vi "LVClass_ClosedLoopSmoothing_GetData.vi"(0 "ClosedLoopSmoothing in":refnum<class "ClosedLoopSmoothing.lvclass">, 11 "error in (no error)":errorcluster) -> (4 "ClosedLoopSmoothing out":refnum<class "ClosedLoopSmoothing.lvclass">, 6 "CLoopSmoothingParams":T1, 15 "error out":errorcluster)   [LabVIEW 2020, in "ClosedLoopSmoothing.lvclass"]
doc: "Get closed loop smoothing parameters.\n\n<B>smoothing_paramsIn</B> : Closed Loop smoothing params object.\n<B>smoothing_paramsOut</B> : Closed Loop smoothing params object.\n<B>low_gain_factor</B> : lowest value for gain factor\n<B>high_gain_factor</B> : highest value for gain factor\n<B>low_amplitude</B> : lowest amplitude value before switching to linear behavior\n<B>high_amplitude</B> : highest amplitude value where linear behavior stops"
uses:
  ClosedLoopSmoothing.lvclass
  ClosedLoopSmoothingParameters.ctl
  ClosedLoopSmoothing.lvclass/ClosedLoopSmoothing.ctl
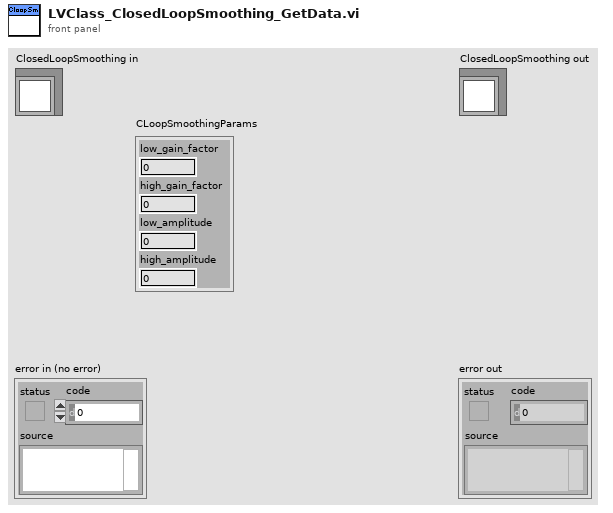
[diagram p1: front panel]
types:
  T1 = typedef "ClosedLoopSmoothingParameters.ctl" = cluster{"low_gain_factor":sgl, "high_gain_factor":sgl, "low_amplitude":i32, "high_amplitude":i32}
  T2 = typedef "ClassID.ctl" = i64
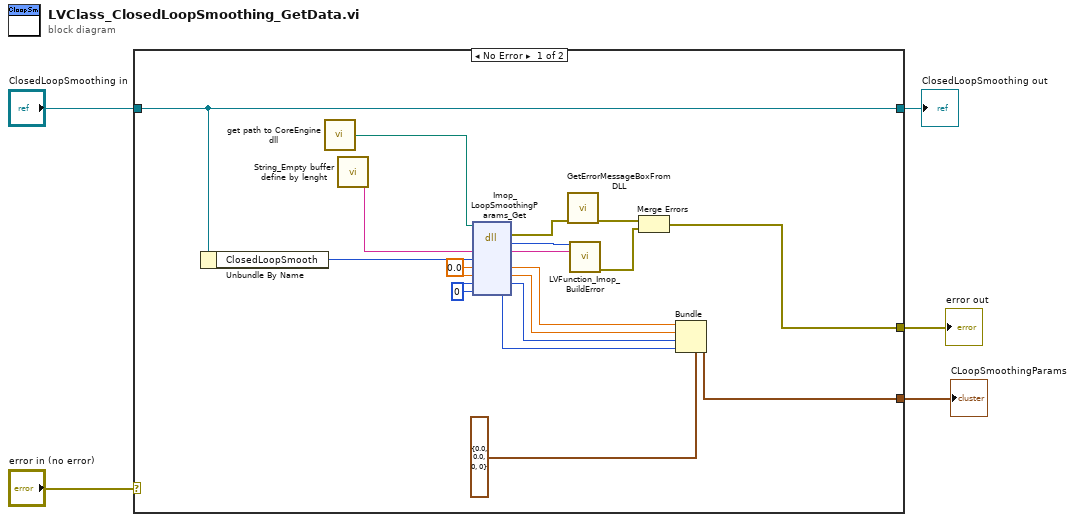
[diagram p0: block diagram]
diagram:
  n1 = case shown="No Error" "error in (no error)" {
    selector: "error in (no error)" -> [_ w25]
    tunnel: [w16 w25] -> w4
    tunnel: [w14 w24] -> w2
    tunnel: "ClosedLoopSmoothing in" -> [w14 w24]
    tunnel: [w8 _] -> w1
    frame No Error {
      w6 = 0 ("High_amplitude")
      w7 = sgl 0.0 ("low_gain_factor")
      n2 = Unbundle By Name(w14) -> ("ClosedLoopSmooth"=w15:T2)
      n3 = call "get path to CoreEngine dll.vi"() -> ("path to wavekit library"=w17:path)  [unwired: 14 in, 1 out]
      n4 = call "String_Empty buffer define by lenght.vi"() -> ("Empty buffer"=w23:string)  [unwired: 1 in]
      n5 = dll-call lib="D:/soft/HASO_v3/SVN_trunk/ImOpCoreEngine4_LV2011/DLLs/c_interface_vc100.dll" fn="Imop_LoopSmoothingParams_Get"(path in=w17, "message"=w23, "smoothing_params"=w15, "low_gain_factor"=w7, "high_gain_factor"=w7, "low_amplitude"=w6, "High_amplitude"=w6) -> (error out=w20:errorcluster, "return type"=w21:i32, "message"=w22:string, "low_gain_factor"=w13:sgl, "high_gain_factor"=w12:sgl, "low_amplitude"=w11:i32, "High_amplitude"=w10:i32)  [unwired: 3 in, 1 out]
      n6 = call "GetErrorMessageBoxFromDLL.vi"("error IN"=w20) -> ("error OUT"=w19:errorcluster)  [unwired: 10 in]
      n7 = call "LVFunction_Imop_BuildError.vi"("code"=w21, "String to Prepend to source (\"\")"=w22) -> ("error out"=w18:errorcluster)  [unwired: 13 in]
      n8 = Merge Errors(w19, w18) -> (w16:errorcluster)
      n9 = Bundle(cluster=T1 {"low_gain_factor"=0.0, "high_gain_factor"=0.0, "low_amplitude"=0, "high_amplitude"=0} ("CLoopSmoothingParams"), "low_gain_factor"=w13, "high_gain_factor"=w12, "low_amplitude"=w11, "high_amplitude"=w10) -> (w8:T1)
    }
    frame Error {
    }
  }
  "error out" <- w4
  "ClosedLoopSmoothing out" <- w2
  "CLoopSmoothingParams" <- w1
